vi "unwrap2D_main.vi"   [LabVIEW 2015]
uses:
  <vilib>/Analysis/baseanly.llb/Real A x B.vi
  <vilib>/Analysis/Matrix/Numeric/Subtract/Subtract - RM,RM.vi
  <vilib>/Analysis/Matrix/Numeric/Add/Add - RM,RM.vi
  <vilib>/Analysis/Matrix/NI_Matrix.lvlib
  <vilib>/Analysis/NI_AALBase.lvlib
types:
  T1 = typedef "NI_Matrix.lvlib/RealMatrix.ctl" = dbl[][]
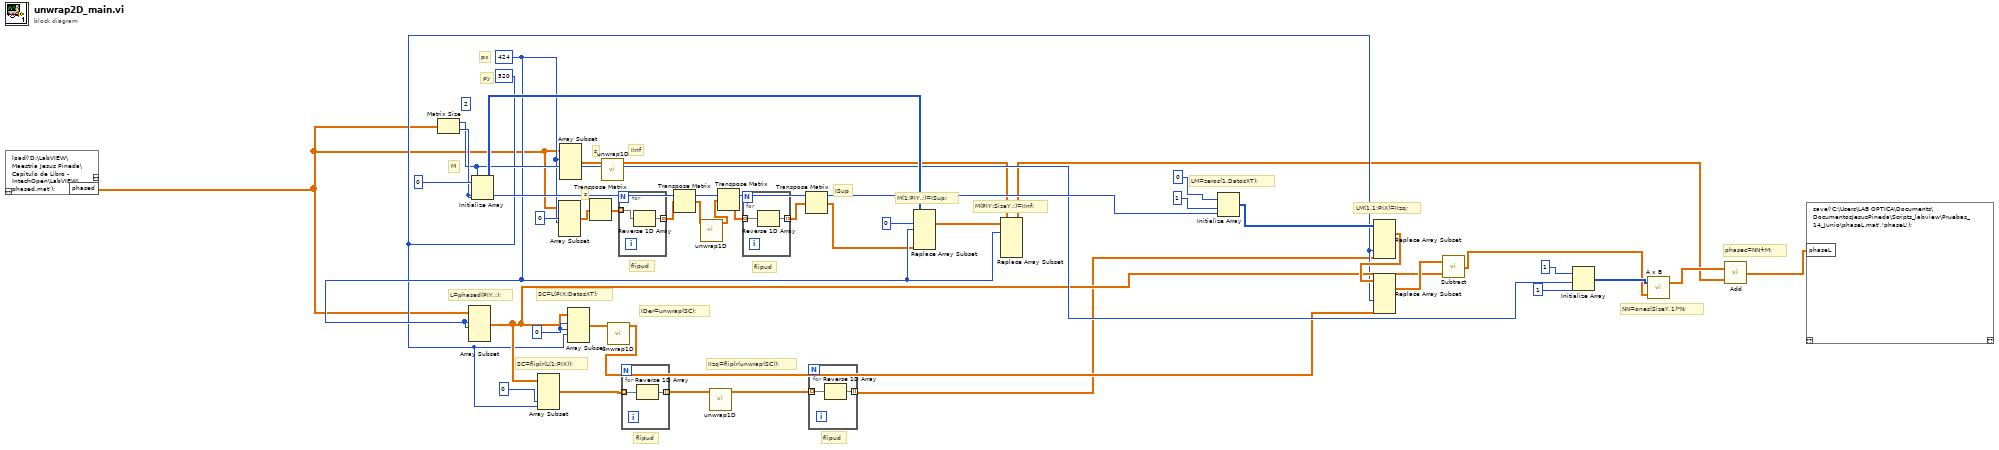
[diagram p0: block diagram]
diagram:
  w9 = 520
  w25 = 424
  w35 = 0
  (unwired) 2
  # "phasec=NN+M;"
  # "NN=ones(SizeY,1)*N;"
  # "py"
  # "IDer=unwrap(SC);"
  # "LM(1,1:PIX)=IIzq;"
  # "LM=zeros(1,DatosXT);"
  # "IIzq=fliplr(unwrap(SC));"
  # "flipud"
  # "SC=fliplr(L(1:PIX));"
  # "flipud"
  # "SC=L(PIX:DatosXT);"
  # "L=phased(PIY,:);"
  # "M(PIY:SizeY,:)=IInf;"
  # "flipud"
  # "M(1:PIY,:)=ISup;"
  # "M"
  # "ISup"
  # "flipud"
  # "s"
  # "s"
  # "IInf"
  # "px"
  n1 = script code="load('D:\\LabVIEW\\Maestria Jesus Pineda\\Capitulo de Libro - IntechOpen\\LabVIEW\\phased.mat');"() -> ("phased"=w3:dbl[][])  [unwired: 1 in, 1 out]
  n2 = Matrix Size(0:w3) -> (1:w28:i32, 2:w32:i32)
  n3 = Array Subset(array=w3, index (row)=w25, length (row)=w25) -> (w12:dbl[][])  [unwired: 2 in]
  n4 = Initialize Array(0, w28, w32) -> (w38:i32[][])
  n5 = Array Subset(array=w12, index (col)=0, length (col)=w9) -> (w11:dbl[][])  [unwired: 2 in]
  n6 = Array Subset(array=w3, index (row)=0, length (row)=w25) -> (w22:dbl[][])  [unwired: 2 in]
  n7 = Array Subset(array=w3, index (row)=w25) -> (w41:dbl[][])  [unwired: 3 in]
  n8 = Array Subset(array=w12, index (row)=w35, length (row)=w35, index (col)=w9) -> (w14:dbl[][])  [unwired: 1 in]
  n9 = Transpose Matrix(1:w22) -> (0:w21:dbl[][])
  n10 = call "unwrap1D.vi"("Array in"=w41) -> ("Array out"=w26:dbl[][])  [unwired: 10 in]
  n11 = call "unwrap1D.vi"("Array in"=w14) -> ("Array out"=w13:dbl[][])  [unwired: 10 in]
  n12 = for {
    tunnel: [w43] -> w24 mode=indexing
    tunnel: w21 -> [w42] mode=indexing
    n13 = Reverse 1D Array(array=w42) -> (reversed array=w43:dbl[])
  }
  n14 = for {
    tunnel: w11 -> [w45] mode=indexing
    tunnel: [w44] -> w8 mode=indexing
    n15 = Reverse 1D Array(array=w45) -> (reversed array=w44:dbl[])
  }
  n16 = Transpose Matrix(1:w24) -> (0:w23:dbl[][])
  n17 = call "unwrap1D.vi"("Array in"=w23) -> ("Array out"=w20:dbl[][])  [unwired: 10 in]
  n18 = call "unwrap1D.vi"("Array in"=w8) -> ("Array out"=w16:dbl[][])  [unwired: 10 in]
  n19 = Transpose Matrix(1:w20) -> (0:w19:dbl[][])
  n20 = for {
    tunnel: w19 -> [w47] mode=indexing
    tunnel: [w46] -> w18 mode=indexing
    n21 = Reverse 1D Array(array=w47) -> (reversed array=w46:dbl[])
  }
  n22 = Transpose Matrix(1:w18) -> (0:w17:dbl[][])
  n23 = for {
    tunnel: w16 -> [w49] mode=indexing
    tunnel: [w48] -> w7 mode=indexing
    n24 = Reverse 1D Array(array=w49) -> (reversed array=w48:dbl[])
  }
  n25 = Replace Array Subset(array=w38, new element=w17, index (dim 0)=0, index (dim 1)=w25) -> (w36:T1)  [unwired: 2 in]
  n26 = Replace Array Subset(array=w36, new element=w26, index (dim 0)=w25) -> (w2:T1)  [unwired: 3 in]
  n27 = Initialize Array(0, 1, w32) -> (w31:i32[][])
  n28 = Replace Array Subset(array=w31, new element=w7, index (dim 3)=w9) -> (w15:T1)  [unwired: 3 in]
  n29 = Replace Array Subset(array=w15, new element=w13, index (dim 2)=w9) -> (w30:T1)  [unwired: 3 in]
  n30 = call-poly <vilib>:"Subtract.vi"("Real Matrix B"=w12, "Real Matrix A"=w30) -> ("A - B"=w4:T1)
  n31 = Initialize Array(1, w28, 1) -> (w5:i32[][])
  n32 = call-poly <vilib>:"A x B.vi"("B"=w4, "A"=w5) -> ("A x B"=w6:T1)  [unwired: 1 out]
  n33 = call-poly <vilib>:"Add.vi"("Real Matrix B"=w2, "Real Matrix A"=w6) -> ("A + B"=w1:T1)
  n34 = script code="save('C:\\Users\\LAB OPTICA\\Documents\\DocumentosJesusPineda\\Scripts_labview\\Pruebas_14_Junio\\phaseL.mat','phaseL');"("phaseL"=w1) -> ()  [unwired: 1 in, 1 out]
